vi "DisableControls.vi"(8 "error in (no error)":errorcluster, 10 "Visible":bool, 11 "Controls":refnum<vi>[](array[refnum])) -> (0 "error out":errorcluster)   [LabVIEW 2019]
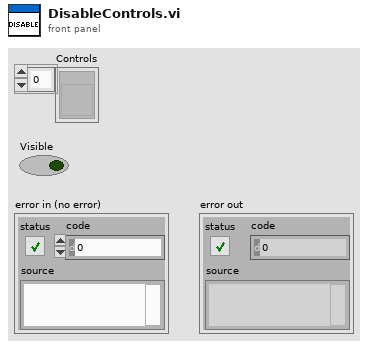
[diagram p1: front panel]
types:
  T1 = enum8{"Enabled", "Disabled", "Disabled and Grayed Out"}
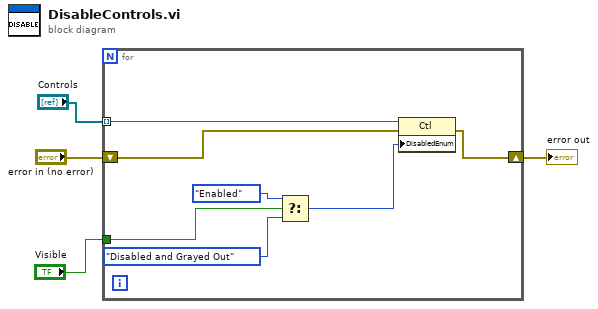
[diagram p0: block diagram]
diagram:
  n1 = for {
    tunnel: "Controls" -> [w11] mode=indexing
    tunnel: "Visible" -> [w8]
    shift-right: [w9] -> w4
    shift-left: "error in (no error)" -> [w10]
    n2 = Select(t=T1."Enabled" ("Disabled"), s=w8, f=T1."Disabled and Grayed Out" ("Disabled")) -> (s? t:f=w5:T1)
    n3 = property class="Ctl"(reference=w11, error in=w10, "DisabledEnum"=w5) -> (error out=w9:errorcluster)  [unwired: 1 out]
  }
  "error out" <- w4
